vi "Read Multi Variant.vi"(8 "error in (no error)":errorcluster, 10 "Tag":string[](array[string]), 11 "Var Bus in":refnum<class "Omni_Bus.lvclass">) -> (0 "error out":errorcluster, 2 "Array":variant[](array[variant]), 3 "Var Bus out":refnum<class "Omni_Bus.lvclass">)   [LabVIEW 2021, in "Omni_Bus.lvclass"]
uses:
  Omni_Bus.lvclass
  Omni_Bus.lvclass/Omni_Bus.ctl
  <vilib>/TSA/Abstract Data Classes/Abs_Types/Variant/Abs_Variant.lvclass
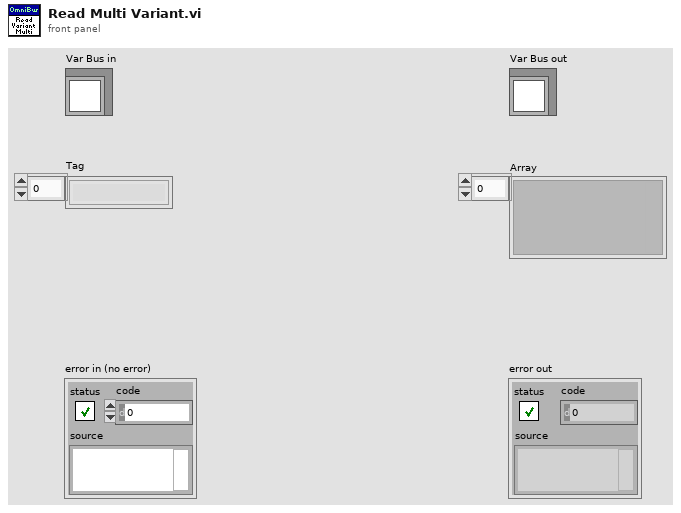
[diagram p1: front panel]
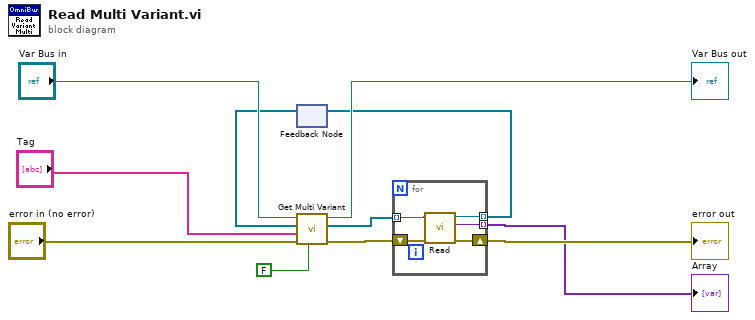
[diagram p0: block diagram]
diagram:
  n1 = feedback #1() -> (w7:refnum<class "Abs_Variant.lvclass">[])  [unwired: 1 in]
  n2 = call-dynamic "Get Multi Variant.vi"("Write?"=FALSE, "error in (no error)"="error in (no error)", "Tag"="Tag", "Value Type"=w7, "Var Bus in"="Var Bus in") -> ("error out"=w6:errorcluster, "Value Out"=w5:refnum<class "Abs_Variant.lvclass">[], "Var Bus out"=→"Var Bus out":refnum<class "Omni_Bus.lvclass">)  [unwired: 4 in]
  n3 = for {
    tunnel: w5 -> [w15] mode=indexing
    tunnel: [w13] -> w3 mode=indexing
    tunnel: [w12] -> w2 mode=indexing
    shift-right: [w14] -> w4
    shift-left: w6 -> [w16]
    n4 = call-dynamic "Read.vi"("error in (no error)"=w16, "Abs_Variant in"=w15) -> ("error out"=w14:errorcluster, "Variant"=w12:variant, "Abs_Variant out"=w13:refnum<class "Abs_Variant.lvclass">)  [unwired: 7 in]
  }
  "error out" <- w4
  "Array" <- w2
  n5 = feedback-in #1(w3) -> ()
